vi "Pipes Example.vi"() -> ()   [LabVIEW 2022 SP3]
uses:
  Pipes.lvlib
panel:
  in  "V4":bool
  in  "V5":bool
  out "P3-2":bool
  out "P9-1":bool
  in  "MFC1":dbl min=0.0 max=10.0 step=0.1 format="%.1f"
  out "P9":bool
  in  "V1":bool
  in  "V2":bool
  in  "V3":bool
  in  "Stop":bool
  out "P1":bool
  out "P1-3":bool
  out "P1-2":bool
  out "P2":bool
  out "P3":bool
  out "P1-4":bool
  # "Instructions:\nRun this VI and toggle the valves to see the pipe colors change accordingly."
  # "Pipes are Classic Flat Square Boolean Indicators, edit the pipe descriptions to\nadd one or more color definitions formatted as:"
  # "Pipe Description Format:\nx<color_hex>|<pipe_name>:[<expression>]"
  # "Expressions supported:\nAND:          and | && | &\nOR:           or | '||' | '|'\nNOT:          not | !\nEQUAL:        ==\nNOT EQUAL:    !=\nLESS THAN:    <\nGREATER THAN: >\nLTE:          <=\nGTE:          >=\nPARENTHESES:  (..)\nLITERAL:      Boolean | DBL | I32 | U32\nIDENTIFIER:   [A-Za-z_][A-Za-z0-9_]*"
  # "If the expression is evaluated to True, the pipe value is set to True and the\ncolor is set to <color_hex> or clone's the <pipe_name> color.\nIf expression is empty, the referenced <pipe_name> value and color are\ncloned (usefull for multi-pipe segments)."
  # "Gas\nInlet"
  # "P1 Description:\nxFF0000:V1 and V2\nxFFA833:V2\nx5B9DF1:V1"
  # "P1-2,3,4 Descriptions:\nP1:"
  # "Water\nInlet"
  # "Example:\nV1 and not V2 and (MFC1 > 4.5 or V3) or V5"
  # "P2 Description:\nP1:P1 and V3"
  # "P3 Description:\nP1:P1 and V4"
  # ">= 0.5"
  # "P9 Description:\nP2:P2 and MFC1 >= 0.5\nP3:P3 and V5"
  # "Outlet"
  # "P9-1 Description:\nP9:"
  # "P3-2 Description:\nP3:"
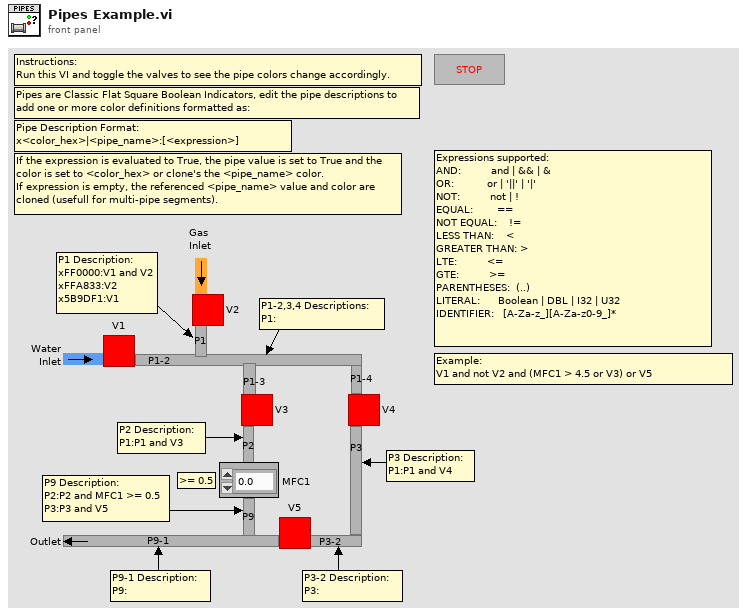
[diagram p1: front panel]
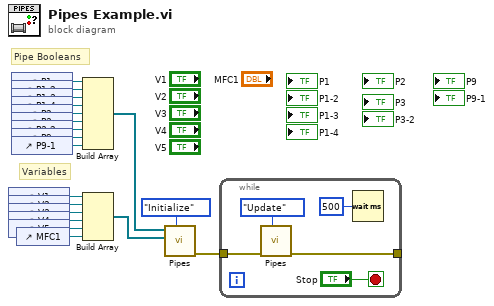
[diagram p0: block diagram]
diagram:
  # "Variables"
  # "Pipe Booleans"
  n1 = control-ref of="V1"() -> (w6:refnum<vi>)
  n2 = control-ref of="V2"() -> (w5:refnum<vi>)
  n3 = control-ref of="V3"() -> (w4:refnum<vi>)
  n4 = control-ref of="V4"() -> (w3:refnum<vi>)
  n5 = control-ref of="V5"() -> (w2:refnum<vi>)
  n6 = control-ref of="P1"() -> (w15:refnum<vi>)
  n7 = control-ref of="P1-2"() -> (w14:refnum<vi>)
  n8 = control-ref of="P1-3"() -> (w13:refnum<vi>)
  n9 = control-ref of="P1-4"() -> (w12:refnum<vi>)
  n10 = control-ref of="P2"() -> (w11:refnum<vi>)
  n11 = control-ref of="P3"() -> (w10:refnum<vi>)
  n12 = control-ref of="P3-2"() -> (w9:refnum<vi>)
  n13 = control-ref of="P9"() -> (w8:refnum<vi>)
  n14 = control-ref of="P9-1"() -> (w7:refnum<vi>)
  n15 = control-ref of="MFC1"() -> (w1:refnum<vi>)
  n16 = Build Array(w15, w14, w13, w12, w11, w10, w9, w8, w7) -> (w17:refnum<vi>[])
  n17 = Build Array(w6, w5, w4, w3, w2, w1) -> (w16:refnum<vi>[])
  n18 = call "Pipes.vi"("Action"=enum16{"Initialize", "Update"}."Initialize", "Variables"=w16, "Pipes"=w17) -> ("error out"=w18:errorcluster)  [unwired: 8 in]
  n19 = while {
    tunnel: w18 -> [w23]
    tunnel: [w21] -> _
    stop <- "Stop" stop-if-true
    n20 = call "Pipes.vi"("Action"=enum16{"Initialize", "Update"}."Update", "error in (no error)"=w23) -> ("error out"=w21:errorcluster)  [unwired: 9 in]
    n21 = Wait (ms)(milliseconds to wait=u32 500) -> ()  [unwired: 1 out]
  }
